vi "Calculate Resistivity Parameters.vi"(0 "ResistData":T2 {"Angles" format="%.6f"; "Voltages" format="%.4f"; "Frequency (Hz)" format="%.1f"; "Rseries (K)" format="%.3f"}, 2 "Print":bool, 5 "2P/4P":bool, 6 "Cell":i32) -> (3 "C13 (pf)":dbl format="%.2f", 4 "R13 (k)":dbl format="%.4f", 7 "Rxg (k)":dbl[](array[numeric]) format="%.4f", 8 "ResistParams":T1 {"C13 (pf)" format="%.2f"; "R13 (k)" format="%.4f"; "C3G (pf)" format="%.2f"; "R3G (k)" format="%.4f"; "C23 (pf)" format="%.2f"; "R23 (k)" format="%.4f"; "C12 (pf)" format="%.2f"; "R12 (k)" format="%.4f"; "C2P (pf)" format="%.2f"; "R2P (k)" format="%.4f"}, 9 "Cxg (pf)":dbl[](array[numeric]) format="%.2f", 10 "Zxg":cdb[](array[numeric]) format="%.6f", 11 "ErrOut":bool, 12 "R2P (k)":dbl format="%.4f", 13 "C3G (pf)":dbl format="%.2f", 14 "C2P (pf)":dbl format="%.2f", 15 "R12 (k)":dbl format="%.4f", 16 "C12 (pf)":dbl format="%.2f", 17 "R23 (k)":dbl format="%.4f", 18 "C23 (pf)":dbl format="%.2f", 19 "R3G (k)":dbl format="%.4f")   [LabVIEW 2013]
doc: "This vi computes the real and reactive components of an idealized rock based on the standard rock model - three series sections where each section consists of a resistor in parallel with a capacitor. All input parameters are supplied via the input cluster 'ResistData' as follows:\n\nResistor - the series dropping resistor in kohms;\nFrequency - the excitation frequency in Khz;\nVoltages - the array of four peak voltages (Vgen, Vtop, Vp1, Vp2) relative to ground;\nAngles - the array of phase angles in degrees of the four voltages relative to Vgen (phase = 0).\n\nThe resistivity parameters are returned in the following variables:\n\nR2P (k) - the two-pole resistance in Kohms (from the top of the rock to ground);\nC2P (pf) - the two-pole capacitance in picofarads (from the top of the rock to ground);\nR12 (k) - the resistance in Kohms between the top of the rock and the 1st point contact;\nC12 (pf) - the capacitance in picofarads between the top of the rock and the 1st point contact;\nR23 (k) - the resistance in Kohms between the 1st and 2nd point contacts;\nC23 (pf) - the capacitance in picofarads between the 1st and 2nd point contacts;\nR3G (k) - the resistance in Kohms between the 2nd point contact and ground;\nC3G (pf) - the capacitance in picofarads between the 2nd point contact and ground;\nErrOut - a Boolean which is TRUE if any of the above 8 values is less than zero (FALSE o.w);\nZxg - the array of 4 impedances to ground representing Zgen, Ztop, Zp1, and Zp2;\nRxg (k) - the array of 4 resistances in Kohms representing the real part of Zgen, Ztop, Zp1,\n and Zp2 to ground;\nCxg (pf) - the array of 4 capacitances in picofarads representing the imaginary part of Zgen\n Ztop, Zp1, and Zp2 to ground;\n\nThe vi is provided with a test mode where the generator voltage and frequency, and the required four resistor and three capacitor values can be input via the front panel. Setting 'Test' fo TRUE will cause the test code to calculate the 'ResistData' cluster and submit this data to the calculation section instead of the data input via the connector. The vi should return the values input via the 'Simxxxxxx' controls.\n\nAutoCon, 7/2000"
uses:
  <vilib>/Utility/NIReport.llb/NI_report.lvclass
panel:
  in  "Enabled":bool=TRUE
  out "AllErrs":bool[](array[boolean])
  in  "ErrEnbl":bool[](array[boolean])=[TRUE, FALSE, TRUE, FALSE, TRUE, FALSE, FALSE, FALSE, TRUE, FALSE]
  out "Text Results":string="      ***   RESISTIVITY TEST RESULTS   ***\r\n\r\nCell #: Cell 2\r\nDate: 7/27/2005\tTime: 11:15 PM\r\n\r\nINPUT DATA\r\n\r\nSeries R (Kohms) = 100.000, \tFreq (Hz) = 1000\r\nVgen = 1.407, \tAngle0 = 0.00\r\nV1g =  0.747, \tAngle1 = -36.83\r\nV2g =  0.421, \tAngle2 = -67.72\r\nV3g =  0.189, \tAngle3 = -90.98\r\n\r\n\r\nRESULTS\r\n\r\nR12 (Kohms) = 59.573, \tC12 (pf) = 1981\r\nR13 (Kohms) = 115.790, \tC13 (pf) = 1777\r\nR14 (Kohms) = 197.439, \tC14 (pf) = 1796\r\nR23 (Kohms) = 159.703, \tC23 (pf) = 5603\r\nR34 (Kohms) = -40.971, \tC34 (pf) = 6735\r\n"
  out "Ix_Calc":cdb format="%.8f"
  out "Ix":cdb format="%.8f"
  out "Ztot":cdb format="%.6f"
  out "Z3G":cdb format="%.6f"
  out "Z23":cdb format="%.6f"
  out "Z12":cdb format="%.6f"
  in  "SimVgen (Vrms)":sgl=1.0 min=0 max=10 format="%.2f"
  in  "SimC3G":sgl=5600.0 min=0 format="%.3f"
  in  "SimC23":sgl=8200.0 min=0 format="%.3f"
  in  "SimC12":sgl=3300.0 min=0 format="%.3f"
  in  "SimR3G":sgl=0.1926 min=0.01 max=100000 format="%.4f"
  in  "SimR23":sgl=0.35 min=0.01 max=100000 format="%.4f"
  in  "SimR12":sgl=0.12 min=0.01 max=100000 format="%.4f"
  in  "SimResistor (K)":sgl=0.243 min=0.1 max=1000 format="%.3f"
  in  "SimFreq (Hz)":sgl=1.0 min=0.1 max=100 format="%.1f"
  in  "Simulate":bool
  # "Resistors (Kohm)"
  # "Capacitors (pf)"
  # "Complex Impedances"
  # "Rock Current & Total Impedance"
  # "R2P  C2P  R12   C12  R23  C23  R3G  C3G  R13  C13"
  # "Rs=0   f=0   R2P  C2P  R12   C12  R23  C23  R3G  C3G  R13  C13"
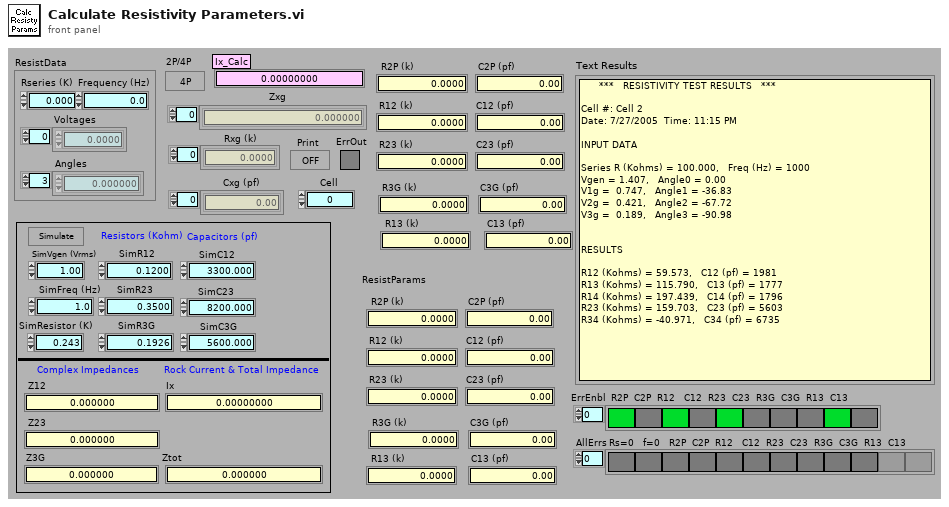
[diagram p1: front panel]
types:
  T1 = cluster{"R2P (k)":dbl, "C2P (pf)":dbl, "R12 (k)":dbl, "C12 (pf)":dbl, "R23 (k)":dbl, "C23 (pf)":dbl, "R3G (k)":dbl, "C3G (pf)":dbl, "R13 (k)":dbl, "C13 (pf)":dbl}
  T2 = cluster{"Rseries (K)":dbl, "Frequency (Hz)":dbl, "Voltages":dbl[], "Angles":dbl[]}
  T3 = cluster{"charset (-1)":i16, "weight (-1)":i16, "name":string, "size":string}
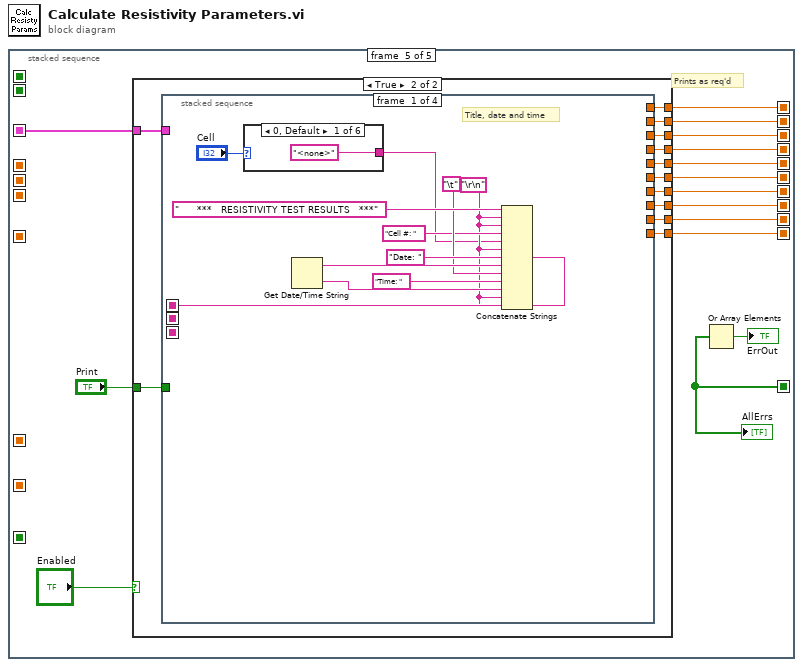
[diagram p0: block diagram]
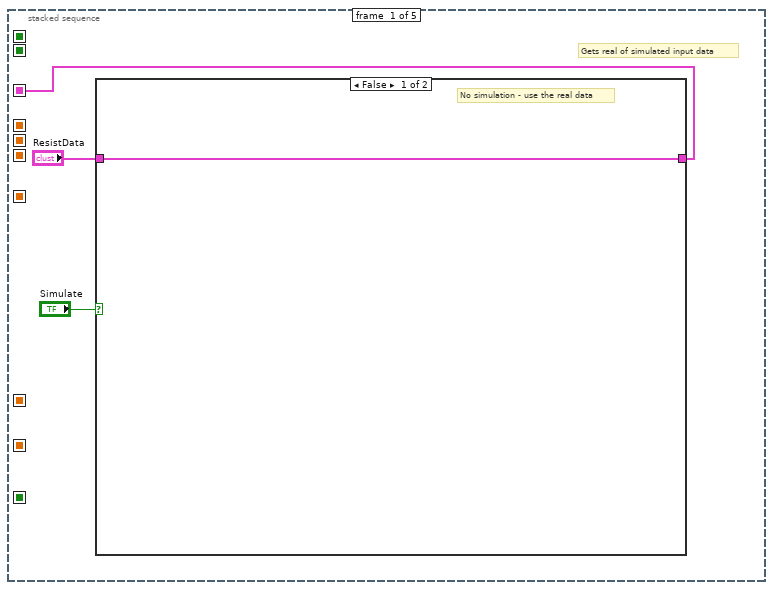
[diagram p2: hidden frame]
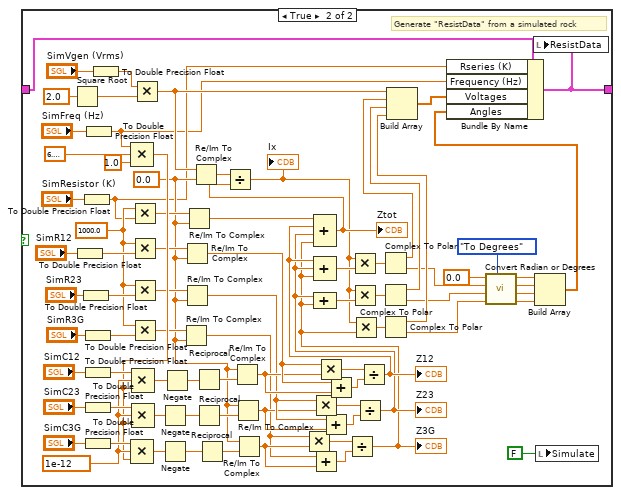
[diagram p3: hidden frame]
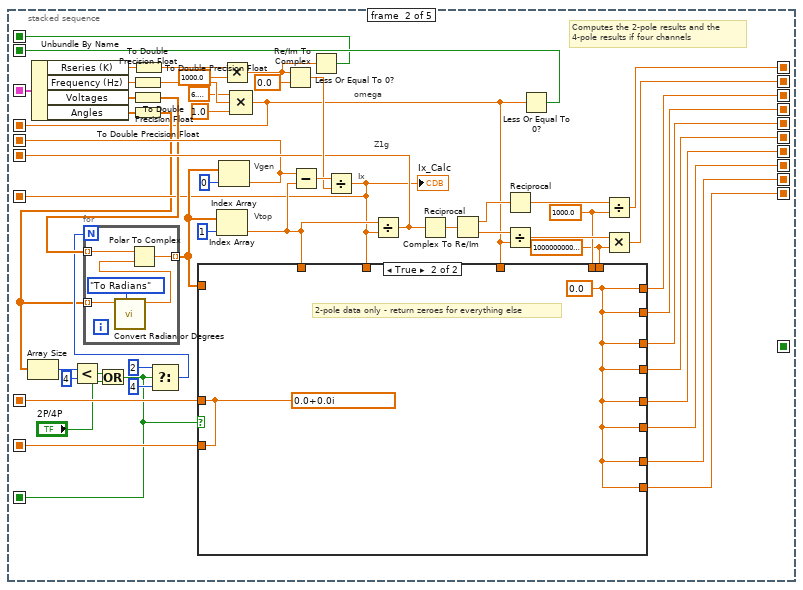
[diagram p4: hidden frame]
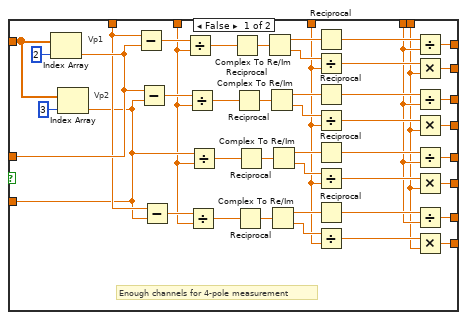
[diagram p5: hidden frame]
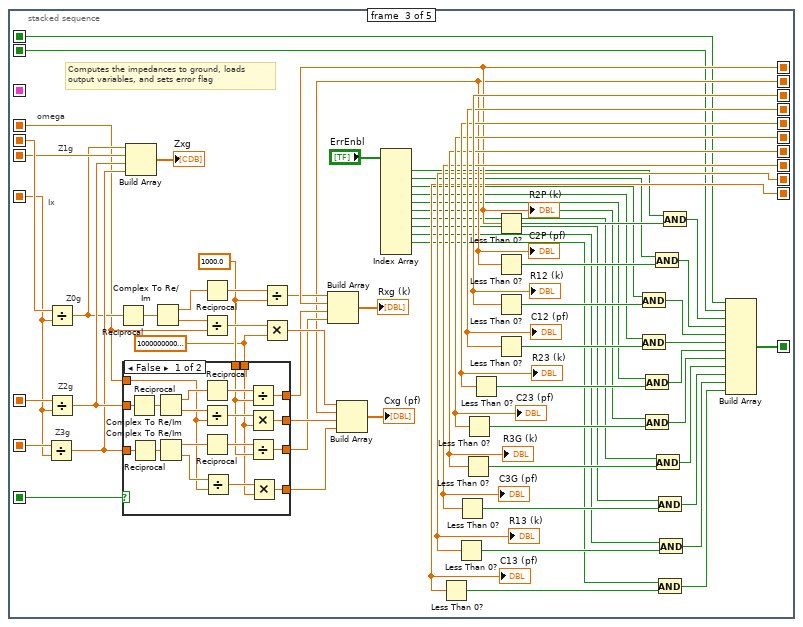
[diagram p6: hidden frame]
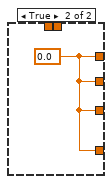
[diagram p7: hidden frame]
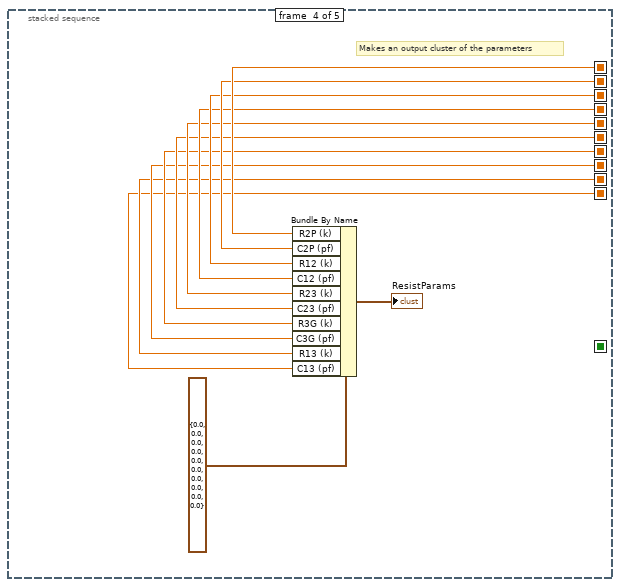
[diagram p8: hidden frame]
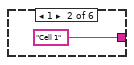
[diagram p10: hidden frame]
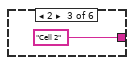
[diagram p11: hidden frame]
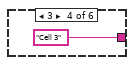
[diagram p12: hidden frame]
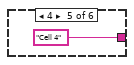
[diagram p13: hidden frame]
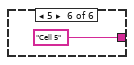
[diagram p14: hidden frame]
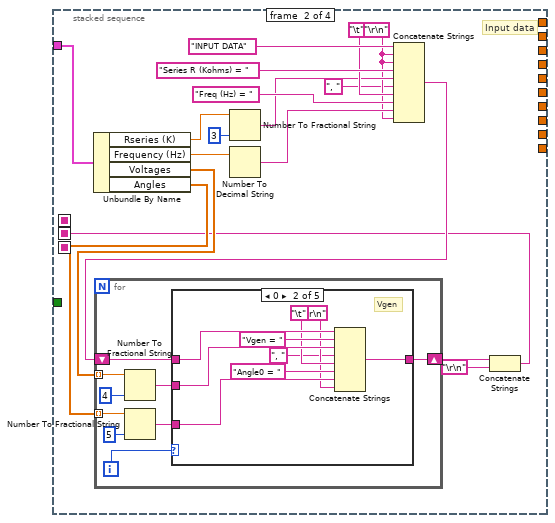
[diagram p15: hidden frame]
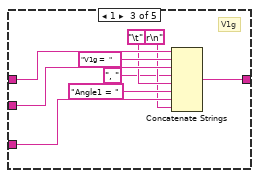
[diagram p17: hidden frame]
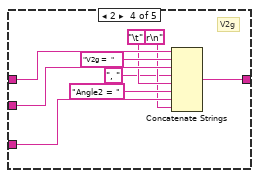
[diagram p18: hidden frame]
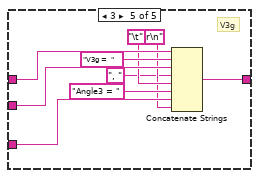
[diagram p19: hidden frame]
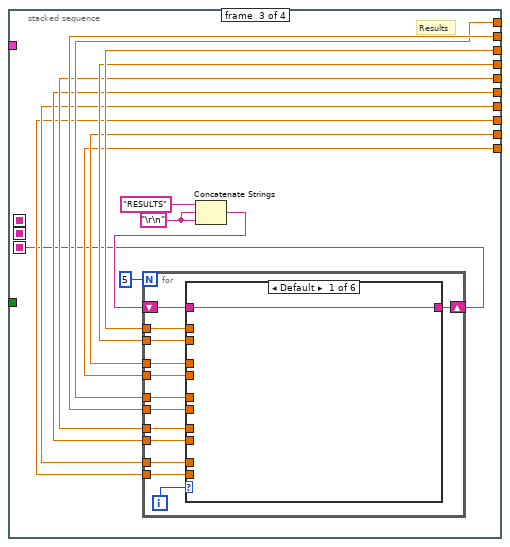
[diagram p20: hidden frame]
diagram:
  n1 = stacked-sequence {
    seq-local: [w1 _ _ _ _] -> [_ w138 _ _ w297]
    seq-local: [_ w108 _ _ _] -> [_ _ w252 _ _]
    seq-local: [_ w120 _ _ _] -> [_ _ w251 _ _]
    seq-local: [_ w119 _ _ _] -> [_ _ w250 _ _]
    seq-local: [_ w118 _ _ _] -> [_ _ w243 w292 w307]
    seq-local: [_ w117 _ _ _] -> [_ _ w228 w291 w306]
    seq-local: [_ w116 _ _ _] -> [_ _ w259 w290 w305]
    seq-local: [_ w115 _ _ _] -> [_ _ w258 w289 w304]
    seq-local: [_ w114 _ _ _] -> [_ _ w257 w288 w303]
    seq-local: [_ w113 _ _ _] -> [_ _ w256 w287 w302]
    seq-local: [_ w112 _ _ _] -> [_ _ w255 w286 w301]
    seq-local: [_ w111 _ _ _] -> [_ _ w254 w285 w300]
    seq-local: [_ w110 _ _ _] -> [_ _ w244 _ _]
    seq-local: [_ w103 _ _ _] -> [_ _ w229 _ _]
    seq-local: [_ w89 _ _ _] -> [_ _ w227 _ _]
    seq-local: [_ w94 _ _ _] -> [_ _ w226 _ _]
    seq-local: [_ w91 _ _ _] -> [_ _ w225 w282 w299]
    seq-local: [_ w90 _ _ _] -> [_ _ w224 w281 w298]
    seq-local: [_ w86 _ _ _] -> [_ _ w192 _ _]
    seq-local: [_ w87 _ _ _] -> [_ _ w193 _ _]
    seq-local: [_ _ w191 _ _] -> [_ _ _ _ w293]
    frame #0 {
      # "Gets real of simulated input data"
      n2 = case shown="False" "Simulate" {
        tunnel: [w4 w65] -> w1
        tunnel: "ResistData" -> [w4 w7]
        frame False {
          # "No simulation - use the real data"
        }
        frame True {
          w20 = 0.0 ("x")
          w79 = 1e-12 ("y")
          w70 = 1000.0 ("y")
          # "Generate \"ResistData\" from a simulated rock"
          n3 = Square Root(x=2.0) -> (sqrt(x)=w47:dbl)
          n4 = To Double Precision Float(number="SimR12") -> (double precision float=w73:dbl)
          n5 = To Double Precision Float(number="SimR23") -> (double precision float=w72:dbl)
          n6 = To Double Precision Float(number="SimResistor (K)") -> (double precision float=w12:dbl)
          n7 = To Double Precision Float(number="SimR3G") -> (double precision float=w71:dbl)
          n8 = To Double Precision Float(number="SimC12") -> (double precision float=w84:dbl)
          n9 = To Double Precision Float(number="SimC23") -> (double precision float=w82:dbl)
          n10 = To Double Precision Float(number="SimC3G") -> (double precision float=w80:dbl)
          n11 = To Double Precision Float(number="SimFreq (Hz)") -> (double precision float=w10:dbl)
          n12 = To Double Precision Float(number="SimVgen (Vrms)") -> (double precision float=w22:dbl)
          n13 = Multiply(x=w70, y=w12) -> (x*y=w50:dbl)
          n14 = Multiply(x=w70, y=w73) -> (x*y=w66:dbl)
          n15 = Multiply(x=w70, y=w72) -> (x*y=w60:dbl)
          n16 = Multiply(x=w70, y=w71) -> (x*y=w59:dbl)
          n17 = Compound Arithmetic op=MULTIPLY(w10, 6.283185307179586, 1.0 ("value")) -> (w78:dbl)
          n18 = Compound Arithmetic op=MULTIPLY(w80, w79, w78) -> (w17:dbl)
          n19 = Multiply(x=w22, y=w47) -> (x*y=w21:dbl)
          n20 = Compound Arithmetic op=MULTIPLY(w84, w79, w78) -> (w19:dbl)
          n21 = Compound Arithmetic op=MULTIPLY(w82, w79, w78) -> (w18:dbl)
          n22 = Negate(x=w18) -> (-x=w15:dbl)
          n23 = Negate(x=w17) -> (-x=w14:dbl)
          n24 = Negate(x=w19) -> (-x=w16:dbl)
          n25 = Re/Im To Complex(1:w20, 2:w59) -> (0:w51:cdb)
          n26 = Re/Im To Complex(1:w20, 2:w66) -> (0:w64:cdb)
          n27 = Re/Im To Complex(1:w20, 2:w60) -> (0:w54:cdb)
          n28 = Re/Im To Complex(1:w20, 2:w50) -> (0:w49:cdb)
          n29 = Re/Im To Complex(1:w20, 2:w21) -> (0:w46:cdb)
          n30 = Reciprocal(x=w16) -> (1/x=w69:dbl)
          n31 = Reciprocal(x=w15) -> (1/x=w68:dbl)
          n32 = Reciprocal(x=w14) -> (1/x=w67:dbl)
          n33 = Re/Im To Complex(1:w69, 2:w20) -> (0:w63:cdb)
          n34 = Re/Im To Complex(1:w68, 2:w20) -> (0:w53:cdb)
          n35 = Re/Im To Complex(1:w67, 2:w20) -> (0:w52:cdb)
          n36 = Multiply(x=w51, y=w52) -> (x*y=w56:cdb)
          n37 = Multiply(x=w54, y=w53) -> (x*y=w58:cdb)
          n38 = Add(x=w51, y=w52) -> (x+y=w55:cdb)
          n39 = Multiply(x=w64, y=w63) -> (x*y=w62:cdb)
          n40 = Add(x=w54, y=w53) -> (x+y=w57:cdb)
          n41 = Add(x=w64, y=w63) -> (x+y=w61:cdb)
          n42 = Divide(x=w56, y=w55) -> (x/y=w32:cdb)
          "Z3G" <- w32
          n43 = Divide(x=w58, y=w57) -> (x/y=w33:cdb)
          "Z23" <- w33
          n44 = Compound Arithmetic op=ADD(w33, w32) -> (w38:cdb)
          n45 = Divide(x=w62, y=w61) -> (x/y=w40:cdb)
          "Z12" <- w40
          n46 = Compound Arithmetic op=ADD(w49, w40, w33, w32) -> (w45:cdb)
          "Ztot" <- w45
          n47 = Divide(x=w46, y=w45) -> (x/y=w36:cdb)
          "Ix" <- w36
          n48 = Compound Arithmetic op=ADD(w40, w33, w32) -> (w44:cdb)
          n49 = Multiply(x=w36, y=w44) -> (x*y=w43:cdb)
          n50 = Multiply(x=w36, y=w38) -> (x*y=w39:cdb)
          n51 = Multiply(x=w36, y=w32) -> (x*y=w35:cdb)
          n52 = Complex To Polar(r * e^(i*theta)=w43) -> (r=w42:dbl, theta=w30:dbl)
          n53 = Complex To Polar(r * e^(i*theta)=w39) -> (r=w37:dbl, theta=w29:dbl)
          n54 = Complex To Polar(r * e^(i*theta)=w35) -> (r=w34:dbl, theta=w28:dbl)
          n55 = Build Array(w21, w42, w37, w34) -> (w9:dbl[])
          n56 = call "Convert Radian or Degrees.vi"("Mode"=enum16{"To Radians", "To Degrees"}."To Degrees", "AngleIn 4"=w28, "AngleIn 3"=w29, "AngleIn 2"=w30, "AngleIn 1"=0.0 ("Input Element")) -> ("AngleOut 4"=w26:dbl, "AngleOut 3"=w25:dbl, "AngleOut 2"=w24:dbl, "AngleOut 1"=w27:dbl)  [unwired: 3 in]
          n57 = Build Array(w27, w24, w25, w26) -> (w8:dbl[])
          n58 = Bundle By Name(cluster=w7, "Rseries (K)"=w12, "Frequency (Hz)"=w10, "Voltages"=w9, "Angles"=w8) -> (w65:T2)
          n59 = local write "ResistData"(w65) -> ()
          n60 = local write "Simulate"(FALSE ("Simulate")) -> ()
        }
      }
    }
    frame #1 {
      w122 = 1000.0 ("y")
      w121 = 1000000000000.0 ("y")
      # "Computes the 2-pole results and the\n4-pole results if four channels"
      # "omega"
      # "Z1g"
      # "Ix"
      # "Vtop"
      # "Vgen"
      n61 = Unbundle By Name(w138) -> ("Rseries (K)"=w137:dbl, "Frequency (Hz)"=w135:dbl, "Voltages"=w107:dbl[], "Angles"=w105:dbl[])
      n62 = To Double Precision Float(number=w135) -> (double precision float=w134:dbl)
      n63 = To Double Precision Float(number=w107) -> (double precision float=w106:dbl[])
      n64 = To Double Precision Float(number=w105) -> (double precision float=w99:dbl[])
      n65 = Array Size(array=w99) -> (size(s)=w98:i32)
      n66 = Less?(x=w98, y=4) -> (x < y?=w96:bool)
      n67 = Or(x=w96, y="2P/4P") -> (x .or. y?=w94:bool)
      n68 = To Double Precision Float(number=w137) -> (double precision float=w136:dbl)
      n69 = Select(t=2, s=w94, f=4) -> (s? t:f=w100:i32)
      n70 = for {
        N: w100 -> [_]
        tunnel: w106 -> [w188] mode=indexing
        tunnel: w99 -> [w190] mode=indexing
        tunnel: [w187] -> w104 mode=indexing
        n71 = call "Convert Radian or Degrees.vi"("Mode"=enum16{"To Radians", "To Degrees"}."To Radians", "AngleIn 1"=w190) -> ("AngleOut 1"=w186:dbl)  [unwired: 6 in, 3 out]
        n72 = Polar To Complex(1:w186, 2:w188) -> (0:w187:cdb)
      }
      n73 = Index Array(array=w104, index=1 ("Index")) -> (element=w109:cdb)
      n74 = Index Array(array=w104, index=0 ("Index")) -> (element=w108:cdb)
      n75 = Multiply(x=w136, y=1000.0) -> (x*y=w88:dbl)
      n76 = Compound Arithmetic op=MULTIPLY(6.283185307179586, w134, 1.0 ("value")) -> (w89:dbl)
      n77 = Re/Im To Complex(1:0.0 ("y"), 2:w88) -> (0:w123:cdb)
      n78 = Subtract(x=w108, y=w109) -> (x-y=w130:cdb)
      n79 = Less Or Equal To 0?(x=w88) -> (x <= 0?=w86:bool)
      n80 = Divide(x=w130, y=w123) -> (x/y=w103:cdb)
      "Ix_Calc" <- w103
      n81 = case shown="True" w94 {
        tunnel: w122 -> [w142 _]
        tunnel: w121 -> [w141 _]
        tunnel: [w161 w185] -> w120
        tunnel: [w152 w185] -> w119
        tunnel: w103 -> [w150 _]
        tunnel: [w160 w184] -> w116
        tunnel: [w159 w184] -> w115
        tunnel: [w158 w184] -> w114
        tunnel: [w157 w184] -> w113
        tunnel: [w156 w184] -> w112
        tunnel: [w155 w184] -> w111
        tunnel: w109 -> [w153 _]
        tunnel: w89 -> [w143 _]
        tunnel: w104 -> [w154 _]
        tunnel: [w140 w184] -> w91
        tunnel: [w139 w184] -> w90
        frame False {
          # "Enough channels for 4-pole measurement"
          # "Vp2"
          # "Vp1"
          n82 = Index Array(array=w154, index=2 ("Index")) -> (element=w161:cdb)
          n83 = Index Array(array=w154, index=3 ("Index")) -> (element=w152:cdb)
          n84 = Subtract(x=w153, y=w161) -> (x-y=w181:cdb)
          n85 = Subtract(x=w161, y=w152) -> (x-y=w174:cdb)
          n86 = Subtract(x=w153, y=w152) -> (x-y=w151:cdb)
          n87 = Divide(x=w181, y=w150) -> (x/y=w179:cdb)
          n88 = Divide(x=w174, y=w150) -> (x/y=w172:cdb)
          n89 = Divide(x=w151, y=w150) -> (x/y=w144:cdb)
          n90 = Divide(x=w152, y=w150) -> (x/y=w166:cdb)
          n91 = Reciprocal(x=w179) -> (1/x=w180:cdb)
          n92 = Reciprocal(x=w172) -> (1/x=w173:cdb)
          n93 = Reciprocal(x=w144) -> (1/x=w149:cdb)
          n94 = Reciprocal(x=w166) -> (1/x=w167:cdb)
          n95 = Complex To Re/Im(x + iy=w180) -> (x=w178:dbl, y=w176:dbl)
          n96 = Complex To Re/Im(x + iy=w173) -> (x=w171:dbl, y=w169:dbl)
          n97 = Complex To Re/Im(x + iy=w149) -> (x=w148:dbl, y=w146:dbl)
          n98 = Complex To Re/Im(x + iy=w167) -> (x=w165:dbl, y=w163:dbl)
          n99 = Reciprocal(x=w178) -> (1/x=w177:dbl)
          n100 = Divide(x=w176, y=w143) -> (x/y=w175:dbl)
          n101 = Reciprocal(x=w171) -> (1/x=w170:dbl)
          n102 = Divide(x=w169, y=w143) -> (x/y=w168:dbl)
          n103 = Reciprocal(x=w165) -> (1/x=w164:dbl)
          n104 = Divide(x=w163, y=w143) -> (x/y=w162:dbl)
          n105 = Reciprocal(x=w148) -> (1/x=w147:dbl)
          n106 = Divide(x=w146, y=w143) -> (x/y=w145:dbl)
          n107 = Divide(x=w177, y=w142) -> (x/y=w160:dbl)
          n108 = Multiply(x=w175, y=w141) -> (x*y=w159:dbl)
          n109 = Divide(x=w170, y=w142) -> (x/y=w158:dbl)
          n110 = Multiply(x=w168, y=w141) -> (x*y=w157:dbl)
          n111 = Divide(x=w164, y=w142) -> (x/y=w156:dbl)
          n112 = Multiply(x=w162, y=w141) -> (x*y=w155:dbl)
          n113 = Divide(x=w147, y=w142) -> (x/y=w140:dbl)
          n114 = Multiply(x=w145, y=w141) -> (x*y=w139:dbl)
        }
        frame True {
          w185 = cdb 0.0+0.0i
          w184 = 0.0
          # "2-pole data only - return zeroes for everything else"
        }
      }
      n115 = Divide(x=w109, y=w103) -> (x/y=w110:cdb)
      n116 = Reciprocal(x=w110) -> (1/x=w127:cdb)
      n117 = Complex To Re/Im(x + iy=w127) -> (x=w125:dbl, y=w126:dbl)
      n118 = Reciprocal(x=w125) -> (1/x=w124:dbl)
      n119 = Divide(x=w126, y=w89) -> (x/y=w129:dbl)
      n120 = Less Or Equal To 0?(x=w89) -> (x <= 0?=w87:bool)
      n121 = Divide(x=w124, y=w122) -> (x/y=w118:dbl)
      n122 = Multiply(x=w129, y=w121) -> (x*y=w117:dbl)
    }
    frame #2 {
      w239 = 1000.0 ("y")
      w238 = 1000000000000.0 ("y")
      # "Computes the impedances to ground, loads\noutput variables, and sets error flag"
      # "Ix"
      # "omega"
      # "Z1g"
      # "Z0g"
      # "Z3g"
      # "Z2g"
      n123 = Divide(x=w250, y=w229) -> (x/y=w248:cdb)
      n124 = Divide(x=w252, y=w229) -> (x/y=w242:cdb)
      n125 = Divide(x=w251, y=w229) -> (x/y=w249:cdb)
      n126 = Reciprocal(x=w242) -> (1/x=w253:cdb)
      n127 = case shown="False" w226 {
        tunnel: w249 -> [w277 _]
        tunnel: w248 -> [w276 _]
        tunnel: w239 -> [w271 _]
        tunnel: w238 -> [w270 _]
        tunnel: [w265 w280] -> w234
        tunnel: [w264 w280] -> w233
        tunnel: [w263 w280] -> w231
        tunnel: [w262 w280] -> w230
        tunnel: w227 -> [w261 _]
        frame False {
          n128 = Reciprocal(x=w277) -> (1/x=w279:cdb)
          n129 = Reciprocal(x=w276) -> (1/x=w278:cdb)
          n130 = Complex To Re/Im(x + iy=w279) -> (x=w269:dbl, y=w268:dbl)
          n131 = Complex To Re/Im(x + iy=w278) -> (x=w267:dbl, y=w266:dbl)
          n132 = Reciprocal(x=w269) -> (1/x=w275:dbl)
          n133 = Divide(x=w268, y=w261) -> (x/y=w274:dbl)
          n134 = Reciprocal(x=w267) -> (1/x=w273:dbl)
          n135 = Divide(x=w266, y=w261) -> (x/y=w272:dbl)
          n136 = Divide(x=w275, y=w271) -> (x/y=w263:dbl)
          n137 = Multiply(x=w274, y=w270) -> (x*y=w265:dbl)
          n138 = Divide(x=w273, y=w271) -> (x/y=w262:dbl)
          n139 = Multiply(x=w272, y=w270) -> (x*y=w264:dbl)
        }
        frame True {
          w280 = 0.0
        }
      }
      n140 = Build Array(w242, w244, w249, w248) -> (→"Zxg":cdb[])
      n141 = Complex To Re/Im(x + iy=w253) -> (x=w237:dbl, y=w236:dbl)
      n142 = Reciprocal(x=w237) -> (1/x=w240:dbl)
      n143 = Divide(x=w236, y=w227) -> (x/y=w241:dbl)
      n144 = Divide(x=w240, y=w239) -> (x/y=w232:dbl)
      n145 = Multiply(x=w241, y=w238) -> (x*y=w235:dbl)
      n146 = Build Array(w232, w243, w231, w230) -> (→"Rxg (k)":dbl[])
      n147 = Build Array(w235, w228, w234, w233) -> (→"Cxg (pf)":dbl[])
      n148 = Index Array(array="ErrEnbl") -> (element #1=w217:bool, element #2=w216:bool, element #3=w213:bool, element #4=w200:bool, element #5=w199:bool, element #6=w198:bool, element #7=w197:bool, element #8=w196:bool, element #9=w195:bool, element #10=w194:bool)  [unwired: 11 in, 1 out]
      n149 = Less Than 0?(x=w224) -> (x < 0?=w202:bool)
      n150 = Less Than 0?(x=w225) -> (x < 0?=w204:bool)
      n151 = Less Than 0?(x=w254) -> (x < 0?=w206:bool)
      n152 = Less Than 0?(x=w255) -> (x < 0?=w223:bool)
      n153 = Less Than 0?(x=w256) -> (x < 0?=w208:bool)
      n154 = Less Than 0?(x=w257) -> (x < 0?=w210:bool)
      n155 = Less Than 0?(x=w243) -> (x < 0?=w260:bool)
      n156 = Less Than 0?(x=w228) -> (x < 0?=w219:bool)
      n157 = Less Than 0?(x=w259) -> (x < 0?=w215:bool)
      n158 = Less Than 0?(x=w258) -> (x < 0?=w212:bool)
      n159 = And(x=w213, y=w215) -> (x .and. y?=w214:bool)
      n160 = And(x=w200, y=w212) -> (x .and. y?=w211:bool)
      n161 = And(x=w199, y=w210) -> (x .and. y?=w209:bool)
      n162 = And(x=w198, y=w208) -> (x .and. y?=w207:bool)
      n163 = And(x=w216, y=w219) -> (x .and. y?=w220:bool)
      n164 = And(x=w197, y=w223) -> (x .and. y?=w222:bool)
      n165 = And(x=w196, y=w206) -> (x .and. y?=w205:bool)
      n166 = And(x=w194, y=w202) -> (x .and. y?=w201:bool)
      n167 = And(x=w195, y=w204) -> (x .and. y?=w203:bool)
      n168 = And(x=w217, y=w260) -> (x .and. y?=w221:bool)
      n169 = Build Array(w192, w193, w221, w220, w214, w211, w209, w207, w222, w205, w203, w201) -> (w191:bool[])
      "R2P (k)" <- w243
      "C2P (pf)" <- w228
      "R12 (k)" <- w259
      "C12 (pf)" <- w258
      "R23 (k)" <- w257
      "C23 (pf)" <- w256
      "R3G (k)" <- w255
      "C3G (pf)" <- w254
      "R13 (k)" <- w225
      "C13 (pf)" <- w224
    }
    frame #3 {
      # "Makes an output cluster of the parameters"
      n170 = Bundle By Name(cluster=T1 {"R2P (k)"=0.0, "C2P (pf)"=0.0, "R12 (k)"=0.0, "C12 (pf)"=0.0, "R23 (k)"=0.0, "C23 (pf)"=0.0, "R3G (k)"=0.0, "C3G (pf)"=0.0, "R13 (k)"=0.0, "C13 (pf)"=0.0} ("ResistParams"), "R2P (k)"=w292, "C2P (pf)"=w291, "R12 (k)"=w290, "C12 (pf)"=w289, "R23 (k)"=w288, "C23 (pf)"=w287, "R3G (k)"=w286, "C3G (pf)"=w285, "R13 (k)"=w282, "C13 (pf)"=w281) -> (→"ResistParams":T1)
    }
    frame #4 {
      # "Prints as req'd"
      n171 = case shown="True" "Enabled" {
        tunnel: w307 -> [_ w314]
        tunnel: w306 -> [_ w313]
        tunnel: w305 -> [_ w318]
        tunnel: w304 -> [_ w317]
        tunnel: w303 -> [_ w312]
        tunnel: w302 -> [_ w311]
        tunnel: w301 -> [_ w310]
        tunnel: w300 -> [_ w309]
        tunnel: w299 -> [_ w316]
        tunnel: w298 -> [_ w315]
        tunnel: w297 -> [_ w319]
        tunnel: "Print" -> [_ w308]
        frame False {
        }
        frame True {
          n172 = stacked-sequence {
            seq-local: [w324 _ _ _] -> [_ _ _ w499]
            seq-local: [_ w339 _ _] -> [_ _ _ w498]
            seq-local: [_ _ w401 _] -> [_ _ _ w497]
            tunnel: w319 -> [_ w354 _ _]
            tunnel: w318 -> [_ _ w414 _]
            tunnel: w317 -> [_ _ w413 _]
            tunnel: w316 -> [_ _ w409 _]
            tunnel: w315 -> [_ _ w408 _]
            tunnel: w314 -> [_ _ w406 _]
            tunnel: w313 -> [_ _ w407 _]
            tunnel: w312 -> [_ _ w405 _]
            tunnel: w311 -> [_ _ w404 _]
            tunnel: w310 -> [_ _ w403 _]
            tunnel: w309 -> [_ _ w402 _]
            tunnel: w308 -> [_ _ _ w495]
            frame #0 {
              w322 = "\r\n"
              # "Title, date and time"
              n173 = case shown="0, Default" "Cell" {
                tunnel: ["<none>" "Cell 1" "Cell 2" "Cell 3" "Cell 4" "Cell 5"] -> w320
                frame 0, Default {
                }
                frame 1 {
                }
                frame 2 {
                }
                frame 3 {
                }
                frame 4 {
                }
                frame 5 {
                }
              }
              n174 = Get Date/Time String() -> (date string=w328:string, time string=w325:string)  [unwired: 3 in]
              n175 = Concatenate Strings("      ***   RESISTIVITY TEST RESULTS   ***" ("string"), w322, w322, "Cell #: " ("string"), w320, w322, "Date: " ("string"), w328, "\t", "Time: " ("string"), w325, w322, w322) -> (w324:string)
            }
            frame #1 {
              w344 = "\r\n"
              # "Input data"
              n176 = Unbundle By Name(w354) -> ("Rseries (K)"=w351:dbl, "Frequency (Hz)"=w346:dbl, "Voltages"=w341:dbl[], "Angles"=w342:dbl[])
              n177 = Number To Fractional String(number=w351, precision (6)=i16 3) -> (F-format string=w347:string)  [unwired: 2 in]
              n178 = Number To Decimal String(number=w346) -> (decimal integer string=w345:string)  [unwired: 1 in]
              n179 = Concatenate Strings("INPUT DATA" ("string"), w344, w344, "Series R (Kohms) = " ("string"), w347, ", " ("string"), "\t", "Freq (Hz) = " ("string"), w345, w344) -> (w343:string)
              n180 = for {
                tunnel: w342 -> [w358] mode=indexing
                tunnel: w341 -> [w363] mode=indexing
                shift-right: [w355] -> w340
                shift-left: w343 -> [w359]
                i -> [w361]
                n181 = Number To Fractional String(number=w363, precision (6)=i16 4) -> (F-format string=w360:string)  [unwired: 2 in]
                n182 = Number To Fractional String(number=w358, precision (6)=i16 5) -> (F-format string=w356:string)  [unwired: 2 in]
                n183 = case shown="0" w361 {
                  tunnel: w360 -> [_ w370 w379 w388 w397]
                  tunnel: w359 -> [w364 w373 w382 w391 w400]
                  tunnel: w356 -> [_ w367 w376 w385 w394]
                  tunnel: [w364 w372 w381 w390 w399] -> w355
                  frame Default {
                  }
                  frame 0 {
                    # "Vgen"
                    n184 = Concatenate Strings(w373, "Vgen = ", w370, ", " ("string"), "\t", "Angle0 = " ("string"), w367, "\r\n") -> (w372:string)
                  }
                  frame 1 {
                    # "V1g"
                    n185 = Concatenate Strings(w382, "V1g =  ", w379, ", " ("string"), "\t", "Angle1 = " ("string"), w376, "\r\n") -> (w381:string)
                  }
                  frame 2 {
                    # "V2g"
                    n186 = Concatenate Strings(w391, "V2g =  ", w388, ", " ("string"), "\t", "Angle2 = " ("string"), w385, "\r\n") -> (w390:string)
                  }
                  frame 3 {
                    # "V3g"
                    n187 = Concatenate Strings(w400, "V3g =  ", w397, ", " ("string"), "\t", "Angle3 = " ("string"), w394, "\r\n") -> (w399:string)
                  }
                }
              }
              n188 = Concatenate Strings(w340, "\r\n") -> (w339:string)
            }
            frame #2 {
              w411 = "\r\n"
              # "Results"
              n189 = Concatenate Strings("RESULTS" ("string"), w411, w411) -> (w410:string)
              n190 = for {
                N: 5 -> [_]
                tunnel: w414 -> [w427]
                tunnel: w413 -> [w426]
                shift-right: [w424] -> w401
                shift-left: w410 -> [w425]
                tunnel: w409 -> [w423]
                tunnel: w408 -> [w422]
                tunnel: w407 -> [w420]
                tunnel: w406 -> [w421]
                tunnel: w405 -> [w419]
                tunnel: w404 -> [w418]
                tunnel: w403 -> [w417]
                tunnel: w402 -> [w416]
                i -> [w428]
                n191 = case shown="Default" w428 {
                  tunnel: w427 -> [_ w438 _ _ _ _]
                  tunnel: w426 -> [_ w432 _ _ _ _]
                  tunnel: w425 -> [w429 w436 w450 w463 w476 w489]
                  tunnel: [w429 w435 w449 w462 w475 w488] -> w424
                  tunnel: w423 -> [_ _ w445 _ _ _]
                  tunnel: w422 -> [_ _ w444 _ _ _]
                  tunnel: w421 -> [_ _ _ w458 _ _]
                  tunnel: w420 -> [_ _ _ w457 _ _]
                  tunnel: w419 -> [_ _ _ _ w471 _]
                  tunnel: w418 -> [_ _ _ _ w470 _]
                  tunnel: w417 -> [_ _ _ _ _ w484]
                  tunnel: w416 -> [_ _ _ _ _ w483]
                  frame Default {
                  }
                  frame 0 {
                    # "R12 & C12"
                    n192 = Number To Fractional String(number=w438, precision (6)=i16 3) -> (F-format string=w434:string)  [unwired: 2 in]
                    n193 = Number To Fractional String(number=w432, precision (6)=i16 0) -> (F-format string=w431:string)  [unwired: 2 in]
                    n194 = Concatenate Strings(w436, "R12 (Kohms) = ", w434, ", " ("string"), "\t", "C12 (pf) = " ("string"), w431, "\r\n") -> (w435:string)
                  }
                  frame 1 {
                    # "R13 & C13"
                    n195 = Number To Fractional String(number=w445, precision (6)=i16 3) -> (F-format string=w448:string)  [unwired: 2 in]
                    n196 = Number To Fractional String(number=w444, precision (6)=i16 0) -> (F-format string=w446:string)  [unwired: 2 in]
                    n197 = Concatenate Strings(w450, "R13 (Kohms) = ", w448, ", " ("string"), "\t", "C13 (pf) = " ("string"), w446, "\r\n") -> (w449:string)
                  }
                  frame 2 {
                    # "R14 & C14 (2P)"
                    n198 = Number To Fractional String(number=w458, precision (6)=i16 3) -> (F-format string=w461:string)  [unwired: 2 in]
                    n199 = Number To Fractional String(number=w457, precision (6)=i16 0) -> (F-format string=w459:string)  [unwired: 2 in]
                    n200 = Concatenate Strings(w463, "R14 (Kohms) = ", w461, ", " ("string"), "\t", "C14 (pf) = " ("string"), w459, "\r\n") -> (w462:string)
                  }
                  frame 3 {
                    # "R23 & C23 (4P)"
                    n201 = Number To Fractional String(number=w471, precision (6)=i16 3) -> (F-format string=w474:string)  [unwired: 2 in]
                    n202 = Number To Fractional String(number=w470, precision (6)=i16 0) -> (F-format string=w472:string)  [unwired: 2 in]
                    n203 = Concatenate Strings(w476, "R23 (Kohms) = ", w474, ", " ("string"), "\t", "C23 (pf) = " ("string"), w472, "\r\n") -> (w475:string)
                  }
                  frame 4 {
                    # "R34 & C34"
                    n204 = Number To Fractional String(number=w484, precision (6)=i16 3) -> (F-format string=w487:string)  [unwired: 2 in]
                    n205 = Number To Fractional String(number=w483, precision (6)=i16 0) -> (F-format string=w485:string)  [unwired: 2 in]
                    n206 = Concatenate Strings(w489, "R34 (Kohms) = ", w487, ", " ("string"), "\t", "C34 (pf) = " ("string"), w485, "\r\n") -> (w488:string)
                  }
                }
              }
            }
            frame #3 {
              n207 = Concatenate Strings(w499, w498, w497) -> (w496:string)
              "Text Results" <- w496
              n208 = case shown="True" w495 {
                tunnel: w496 -> [_ w503]
                frame False {
                }
                frame True {
                  w501 = T3 {"charset (-1)"=-1, "weight (-1)"=-1, "name"="Courier New", "size"="14 "}  # font settings
                  n209 = call <vilib>:"Easy Text Report.vi"("text to be printed"=w503, "font settings"=w501, "report type (Standard)"=enum16{"Standard Report", "HTML"}."Standard Report" ("report type")) -> ("error out"=w500:errorcluster)  [unwired: 12 in]
                  n210 = call <vilib>:"Simple Error Handler.vi"("error in (no error)"=w500) -> ()  [unwired: 4 in, 5 out]
                }
              }
            }
          }
        }
      }
      n211 = Or Array Elements(Boolean array=w293) -> (logical OR=→"ErrOut":bool)
      "AllErrs" <- w293
    }
  }
